vi "Target_Spec_To_I2C.vi"(0 "Input_Data":T1 {"Target_Address" format="%x"; "Target_Type" items=["10 Bit Address", "7 Bit Address"]; "T_On (uS)" min=1e-06; "T_Off (uS)" min=1e-06}) -> (4 "I2C_Data":T3 {"Target_Type" items=["10 Bit Address", "7 Bit Address"]; "Selected_Register_Address" format="%x"; "Target_Address" format="%x"})   [LabVIEW 2023]
doc: "Used to convert the target spec to I2C data"
uses:
  Controls/I2C_Data.ctl
  Controls/Customized_Ring.ctl
  Controls/Add_Target_Specification_.ctl
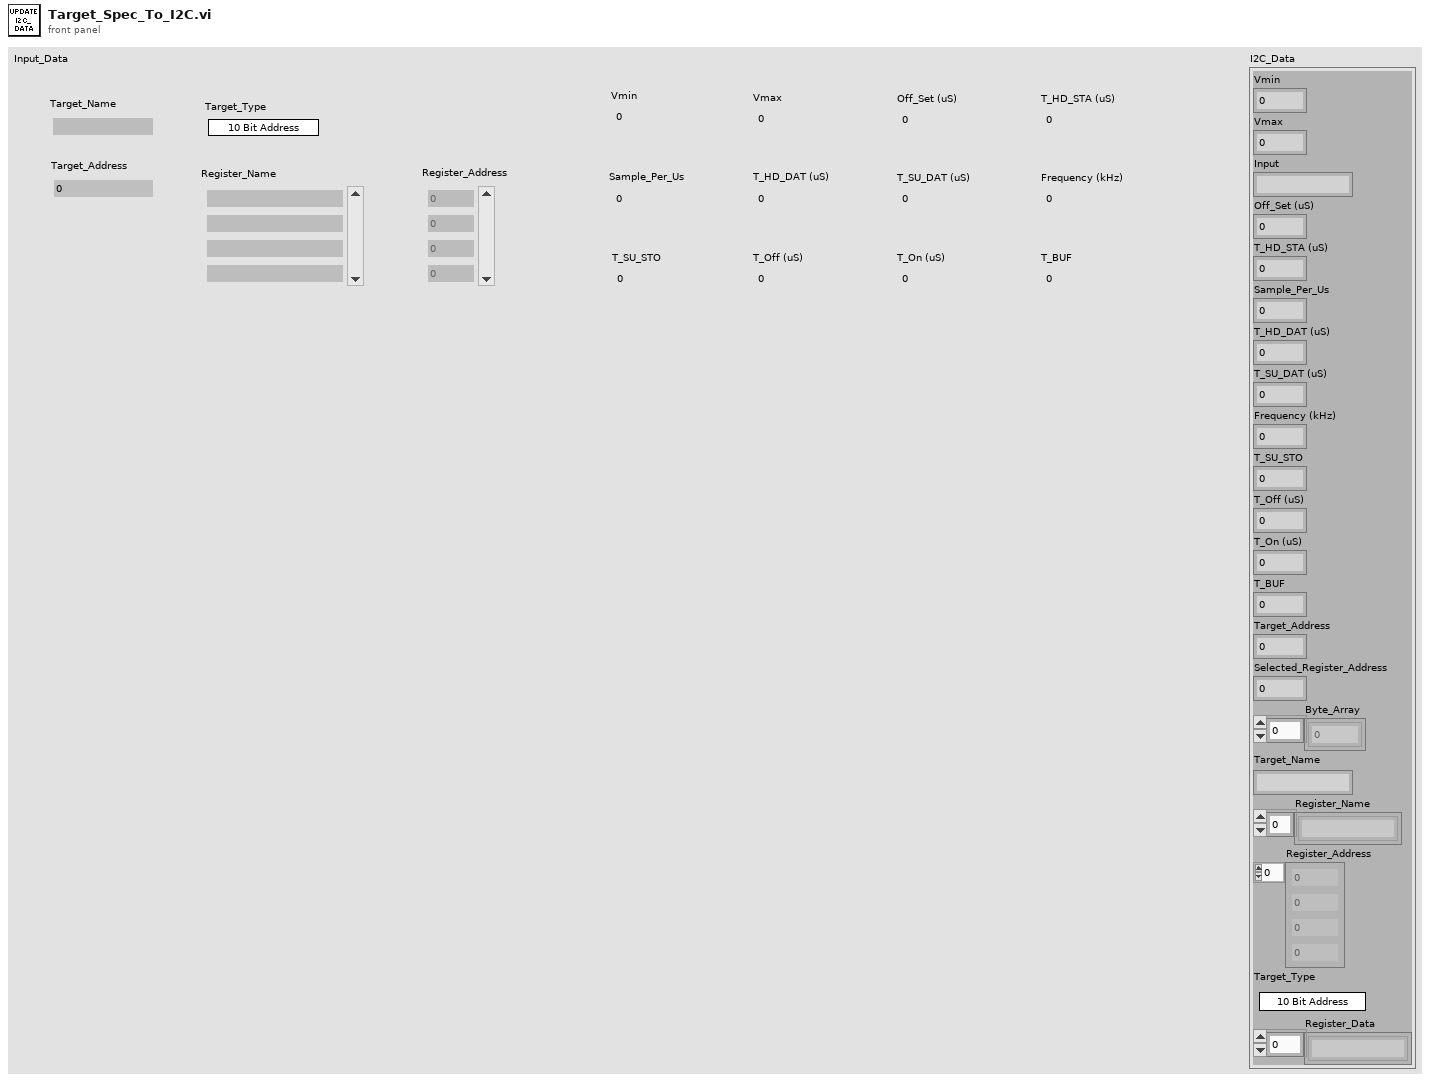
[diagram p1: front panel]
types:
  T1 = typedef "Add_Target_Specification_.ctl" = cluster{"Target_Name":string, "Register_Name":string[], "Register_Address":u16[], "Vmin":dbl, "Vmax":dbl, "Off_Set (uS)":dbl, "T_HD_STA (uS)":dbl, "T_HD_DAT (uS)":dbl, "T_SU_DAT (uS)":dbl, "Frequency (kHz)":dbl, "T_SU_STO":dbl, "T_Off (uS)":dbl, "T_On (uS)":dbl, "T_BUF":dbl, "Sample_Per_Us":dbl, "Target_Type":T2, "Target_Address":u16}
  T2 = typedef "Customized_Ring.ctl" = u16
  T3 = typedef "I2C_Data.ctl" = cluster{"Vmin":dbl, "Vmax":dbl, "Input":string, "Off_Set (uS)":dbl, "T_HD_STA (uS)":dbl, "Sample_Per_Us":dbl, "T_HD_DAT (uS)":dbl, "T_SU_DAT (uS)":dbl, "Frequency (kHz)":dbl, "T_SU_STO":dbl, "T_Off (uS)":dbl, "T_On (uS)":dbl, "T_BUF":dbl, "Target_Address":u16, "Selected_Register_Address":u8, "Byte_Array":u8[], "Target_Name":string, "Register_Name":string[], "Register_Address":u8[], "Target_Type":T2, "Register_Data":string[]}
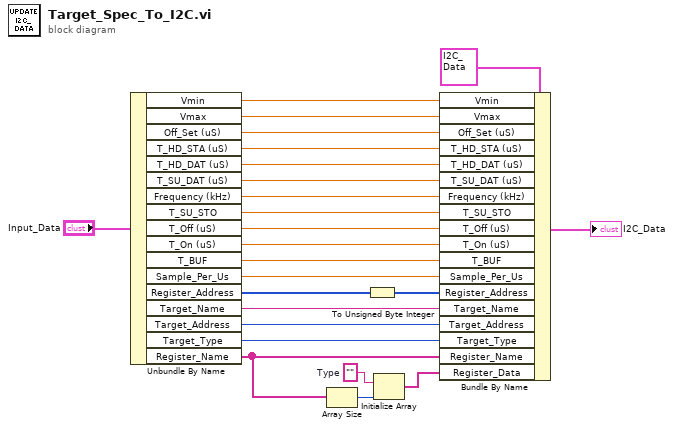
[diagram p0: block diagram]
diagram:
  w3 = ""  # Type
  n1 = Unbundle By Name("Input_Data") -> ("Vmin"=w24:dbl, "Vmax"=w20:dbl, "Off_Set (uS)"=w19:dbl, "T_HD_STA (uS)"=w18:dbl, "T_HD_DAT (uS)"=w17:dbl, "T_SU_DAT (uS)"=w16:dbl, "Frequency (kHz)"=w15:dbl, "T_SU_STO"=w14:dbl, "T_Off (uS)"=w13:dbl, "T_On (uS)"=w12:dbl, "T_BUF"=w11:dbl, "Sample_Per_Us"=w10:dbl, "Register_Address"=w6:u16[], "Target_Name"=w9:string, "Target_Address"=w8:u16, "Target_Type"=w7:T2, "Register_Name"=w2:string[])
  n2 = Array Size(array=w2) -> (size(s)=w4:i32)
  n3 = To Unsigned Byte Integer(number=w6) -> (unsigned 8bit integer=w5:u8[])
  n4 = Initialize Array(w3, w4) -> (w1:string[])
  n5 = Bundle By Name(cluster=T3 {"Vmin"=0.0, "Vmax"=1.0, "Input"="", "Off_Set (uS)"=0.0, "T_HD_STA (uS)"=0.0, "Sample_Per_Us"=0.0, "T_HD_DAT (uS)"=0.0, "T_SU_DAT (uS)"=0.0, "Frequency (kHz)"=0.0, "T_SU_STO"=0.0, "T_Off (uS)"=0.0, "T_On (uS)"=0.0, "T_BUF"=0.0, "Target_Address"=0, "Selected_Register_Address"=0, "Byte_Array"=[], "Target_Name"="", "Register_Name"=[], "Register_Address"=[], "Target_Type"=0, "Register_Data"=[]} ("I2C_Data"), "Vmin"=w24, "Vmax"=w20, "Off_Set (uS)"=w19, "T_HD_STA (uS)"=w18, "T_HD_DAT (uS)"=w17, "T_SU_DAT (uS)"=w16, "Frequency (kHz)"=w15, "T_SU_STO"=w14, "T_Off (uS)"=w13, "T_On (uS)"=w12, "T_BUF"=w11, "Sample_Per_Us"=w10, "Register_Address"=w5, "Target_Name"=w9, "Target_Address"=w8, "Target_Type"=w7, "Register_Name"=w2, "Register_Data"=w1) -> (→"I2C_Data":T3)
